vi "Configure OVP.vi"(7 "Enable OVP (T: Enable)":bool=TRUE, 8 "error in (no error)":errorcluster, 9 "Voltage Limit (0.0 V)":dbl format="%.3g", 11 "VISA resource name":refnum<visa-resource-name>) -> (0 "error out":errorcluster, 3 "VISA resource name out":refnum<visa-resource-name>)   [LabVIEW 2015, in "Agilent E363X Series.lvlib"]
doc: "Configures the power supply's over voltage protection. Specify the over-voltage limit and whether to enable or disable this over voltage protection.\n\n<B>Note:</B> OVP not supported on E3631"
uses:
  Agilent E363X Series.lvlib
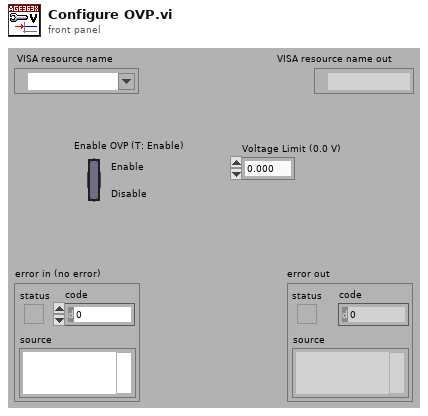
[diagram p1: front panel]
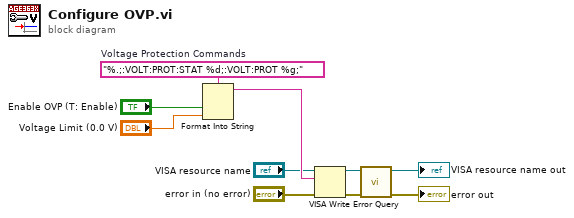
[diagram p0: block diagram]
diagram:
  w8 = "%.;:VOLT:PROT:STAT %d;:VOLT:PROT %g;"  # Voltage Protection Commands
  n1 = Format Into String(format string=w8, "Enable OVP (T: Enable)", "Voltage Limit (0.0 V)") -> (resulting string=w5:string)  [unwired: 2 in, 1 out]
  n2 = VISA Write(VISA resource name="VISA resource name", write buffer=w5, error in (no error)="error in (no error)") -> (VISA resource name out=w6:refnum<visa-resource-name>, error out=w7:errorcluster)  [unwired: 1 out]
  n3 = call "Error Query.vi"("error in (no error)"=w7, "VISA resource name"=w6) -> ("error out"=→"error out":errorcluster, "VISA resource name out"=→"VISA resource name out":refnum<visa-resource-name>)  [unwired: 6 in, 2 out]
